vi "RemoveObserver.vi"(0 "reference in":refnum<class "WeatherStation.lvclass">, 2 "Observer":refnum<class "Observer.lvclass">, 5 "error in (no error)":errorcluster) -> (14 "reference out":refnum<class "WeatherStation.lvclass">, 16 "Removed?":bool, 19 "error out":errorcluster)   [LabVIEW 2010, in "WeatherStation.lvclass"]
uses:
  WeatherStation.lvclass
  Observer_class/Observer.lvclass
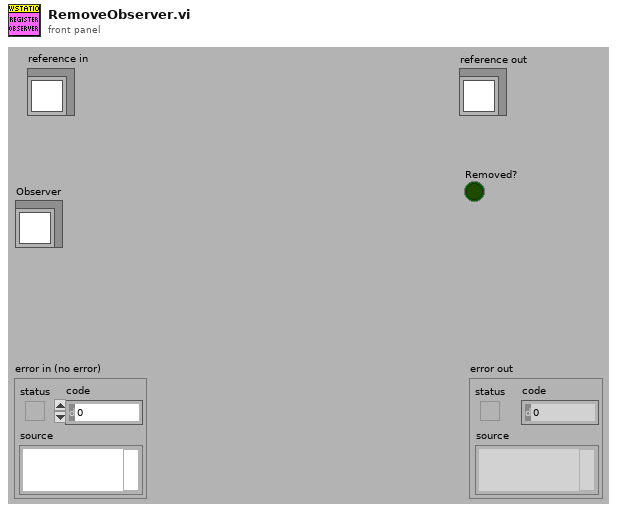
[diagram p1: front panel]
types:
  T1 = typedef "WeatherStation.lvclass/ObjectAttributes.ctl" = cluster{"WeatherData":T2, "Observers":refnum<class "Observer.lvclass">[]}
  T2 = typedef "WeatherData.ctl" = cluster{"Temperature C":dbl, "Humid %":dbl, "Pressure":dbl, "Forecast":string}
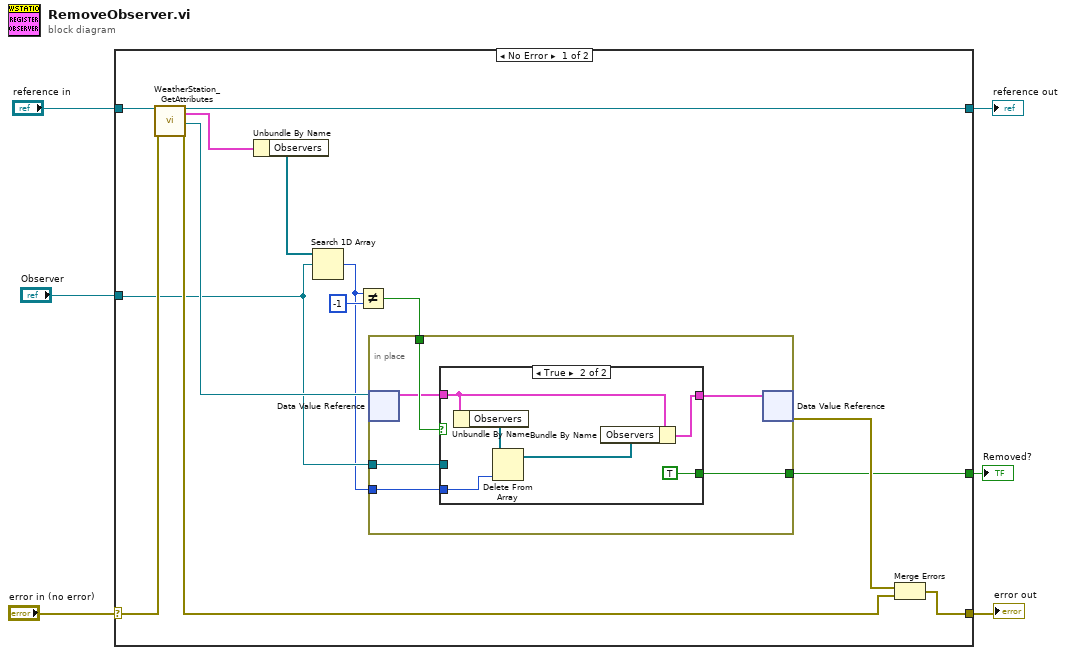
[diagram p0: block diagram]
diagram:
  n1 = case shown="No Error" "error in (no error)" {
    selector: "error in (no error)" -> [w20 w35]
    tunnel: [w13 w35] -> w5
    tunnel: [w17 w34] -> w3
    tunnel: "reference in" -> [w18 w34]
    tunnel: "Observer" -> [w9 _]
    tunnel: [w7 _] -> w1
    frame No Error {
      n2 = call "WeatherStation_GetAttributes.vi"("reference in"=w18, "error in (no error)"=w20) -> ("reference out"=w17:refnum<class "WeatherStation.lvclass">, "Data"=w19:T1, "DataRef"=w11:refnum<data-value>, "error out"=w14:errorcluster)  [unwired: 14 in]
      n3 = Unbundle By Name(w19) -> ("Observers"=w10:refnum<class "Observer.lvclass">[])
      n4 = Search 1D Array(1D array=w10, element=w9) -> (index of element=w8:i32)  [unwired: 1 in]
      n5 = Not Equal?(x=w8, y=-1) -> (x != y?=w12:bool)
      n6 = in-place {
        in-place-border: w12 -> [w26]
        in-place-border: w9 -> [w24]
        in-place-border: w8 -> [w22]
        in-place-border: [w21] -> w7
        n7 = in-place-dvr #1(w11) -> (w25:T1)  [unwired: 1 out]
        n8 = case shown="True" w26 {
          tunnel: w25 -> [w27 w29]
          tunnel: w24 -> [_ _]
          tunnel: [w27 w33] -> w23
          tunnel: w22 -> [_ w32]
          tunnel: [_ TRUE] -> w21
          frame False {
          }
          frame True {
            n9 = Unbundle By Name(w29) -> ("Observers"=w28:refnum<class "Observer.lvclass">[])
            n10 = Delete From Array(array=w28, index=w32) -> (array with subset deleted=w31:refnum<class "Observer.lvclass">[])  [unwired: 1 in, 1 out]
            n11 = Bundle By Name(cluster=w29, "Observers"=w31) -> (w33:T1)
          }
        }
        n12 = in-place-dvr #1(w23) -> (w15:errorcluster)  [unwired: 1 out]
      }
      n13 = Merge Errors(w15, w14) -> (w13:errorcluster)
    }
    frame Error {
    }
  }
  "error out" <- w5
  "reference out" <- w3
  "Removed?" <- w1
